vi "Database_FGV.vi"(8 "error in (no error)":errorcluster, 10 "Write DB Data":T1, 11 "DB Control":T3=enum."Open") -> (0 "error out":errorcluster, 3 "DB Data Out":T1)   [LabVIEW 2013]
doc: "The Database FGV provides access to the file/DB components, manages reads and writes, and provides default data when the file/DB is not available."
uses:
  DB_Data.ctl
  Error Handler/Error_Control.ctl
  Controller/Hardware_Enum.ctl
  DB_control.ctl
panel:
  # "[Covers: CD1A]"
  # "[Covers: CD1B]"
  # "[Covers: CD1C]"
  # "[Covers: CD1D]"
  # "Used for Hardware change over"
  # "[Covers: CD1A]"
  # "[Covers: CD1B]"
  # "[Covers: CD1C]"
  # "[Covers: CD1D]"
  # "Used for Hardware change over"
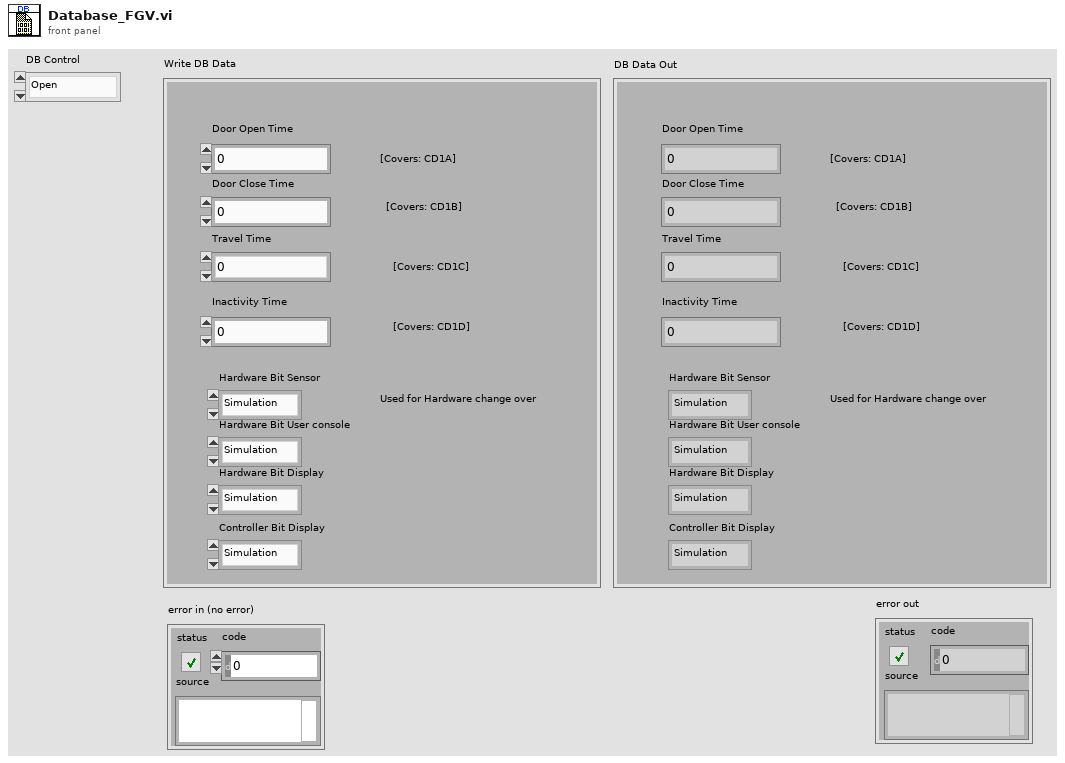
[diagram p1: front panel]
types:
  T1 = typedef "DB_Data.ctl" = cluster{"Door Open Time":dbl, "Travel Time":dbl, "Inactivity Time":dbl, "Door Close Time ":dbl, "Hardware Bit Sensor":T2, "Hardware Bit User console":T2, "Hardware Bit Display":T2, "Controller Bit Display":T2}
  T2 = typedef "Hardware_Enum.ctl" = enum16{"Simulation", "Hardware"}
  T3 = typedef "DB_control.ctl" = enum16{"Initi_FGV", "Open", "Get_Data", "Write_Data", "Write_File", "Close_File"}
  T4 = typedef "Error_Control.ctl" = enum16{"Init", "Console_err", "Process_err", "Sensor_err"}
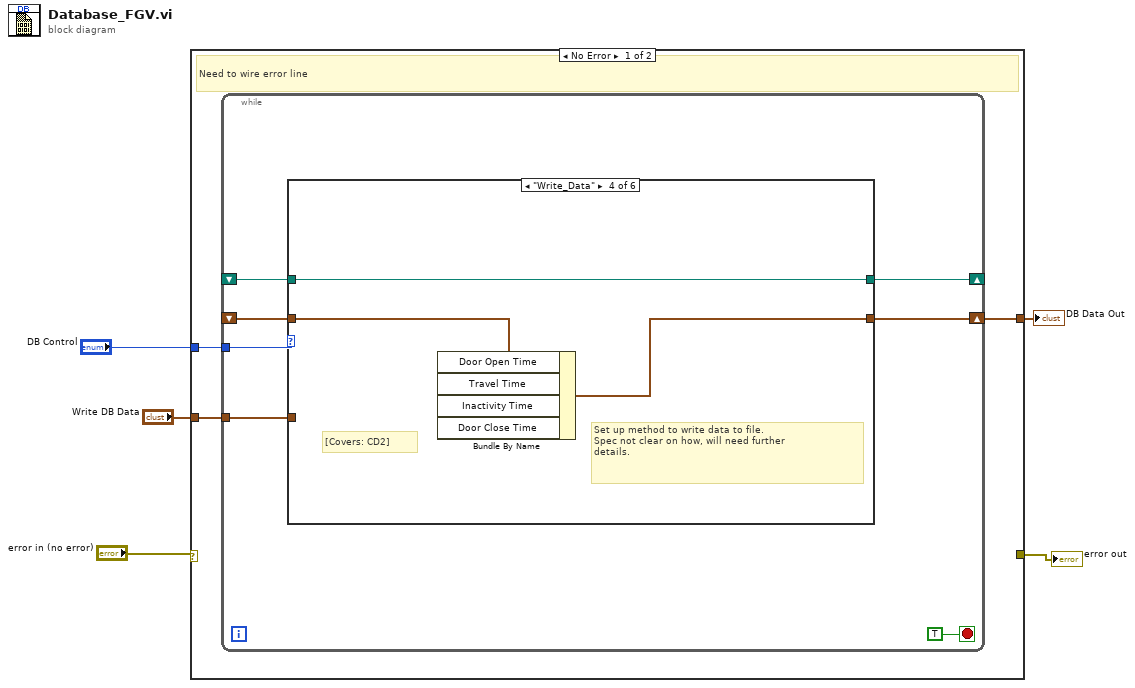
[diagram p0: block diagram]
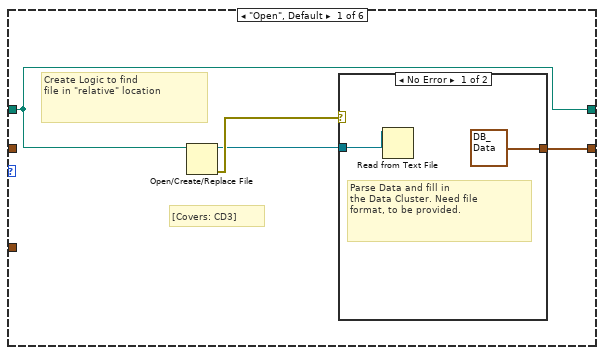
[diagram p2: hidden frame]
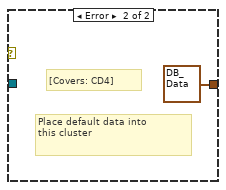
[diagram p3: hidden frame]
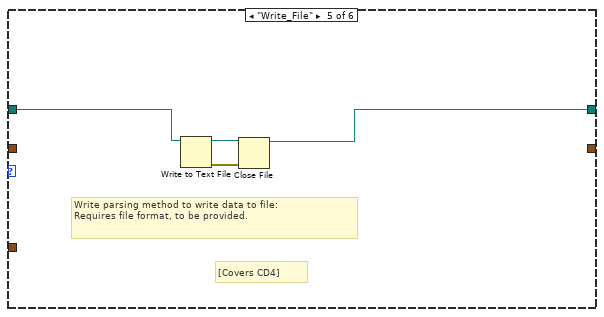
[diagram p6: hidden frame]
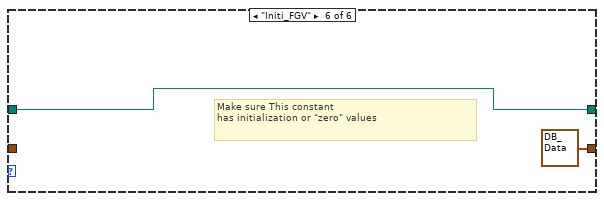
[diagram p7: hidden frame]
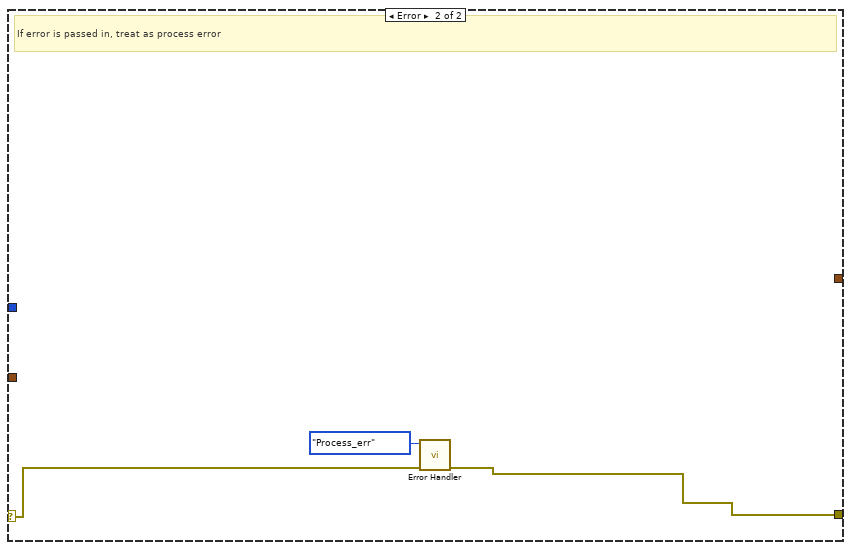
[diagram p8: hidden frame]
diagram:
  n1 = case shown="No Error" "error in (no error)" {
    selector: "error in (no error)" -> [_ w37]
    tunnel: "DB Control" -> [w8 _]
    tunnel: "Write DB Data" -> [w7 _]
    tunnel: [_ w36] -> w2
    tunnel: [w6 _] -> w1
    frame No Error {
      # "Need to wire error line"
      n2 = while {
        tunnel: w8 -> [w14]
        shift-right: [w12] -> w6
        shift-left: _ -> [w11]
        tunnel: w7 -> [w10]
        shift-right: [w9] -> _
        shift-left: _ -> [w13]
        stop <- TRUE stop-if-true
        n3 = case shown="\"Write_Data\"" w14 {
          tunnel: w13 -> [w19 w23 w24 w26 w30 w33]
          tunnel: [w16 _ w25 w27 _ T1 {"Door Open Time"=0.0, "Travel Time"=0.0, "Inactivity Time"=0.0, "Door Close Time "=0.0, "Hardware Bit Sensor"=enum."Simulation", "Hardware Bit User console"=enum."Simulation", "Hardware Bit Display"=enum."Simulation", "Controller Bit Display"=enum."Simulation"} ("DB Data")] -> w12
          tunnel: w11 -> [_ _ w25 w28 _ _]
          tunnel: w10 -> [_ _ _ _ _ _]
          tunnel: [w19 w23 w24 w26 w29 w33] -> w9
          frame "Open", Default {
            # "Create Logic to find\nfile in \"relative\" location"
            # "[Covers: CD3]"
            n4 = Open/Create/Replace File(file path (use dialog)=w19) -> (refnum out=w17:refnum<file>, error out=w18:errorcluster)  [unwired: 5 in, 1 out]
            n5 = case shown="No Error" w18 {
              tunnel: w17 -> [w21 _]
              tunnel: [T1 {"Door Open Time"=0.0, "Travel Time"=0.0, "Inactivity Time"=0.0, "Door Close Time "=0.0, "Hardware Bit Sensor"=enum."Simulation", "Hardware Bit User console"=enum."Simulation", "Hardware Bit Display"=enum."Simulation", "Controller Bit Display"=enum."Simulation"} ("DB Data") T1 {"Door Open Time"=0.0, "Travel Time"=0.0, "Inactivity Time"=0.0, "Door Close Time "=0.0, "Hardware Bit Sensor"=enum."Simulation", "Hardware Bit User console"=enum."Simulation", "Hardware Bit Display"=enum."Simulation", "Controller Bit Display"=enum."Simulation"} ("DB Data")] -> w16
              frame No Error {
                # "Parse Data and fill in \nthe Data Cluster. Need file \nformat, to be provided."
                n6 = Read from Text File(file (use dialog)=w21) -> ()  [unwired: 3 in, 4 out]
              }
              frame Error {
                # "[Covers: CD4]"
                # "Place default data into\nthis cluster"
              }
            }
          }
          frame "Close_File" {
            # "Close file here."
          }
          frame "Get_Data" {
            # "Just pass data for read."
            # "[Covers: CD4]"
          }
          frame "Write_Data" {
            # "Set up method to write data to file.  \nSpec not clear on how, will need further \ndetails."
            # "[Covers: CD2]"
            n7 = Bundle By Name(cluster=w28) -> (w27:T1)  [unwired: 4 in]
          }
          frame "Write_File" {
            # "[Covers CD4]"
            # "Write parsing method to write data to file:\nRequires file format, to be provided."
            n8 = Write to Text File(file (use dialog)=w30) -> (refnum out=w31:refnum<file>, error out=w32:errorcluster)  [unwired: 3 in, 1 out]
            n9 = Close File(refnum=w31, error in=w32) -> (path=w29:path)  [unwired: 1 out]
          }
          frame "Initi_FGV" {
            # "Make sure This constant \nhas initialization or \"zero\" values"
          }
        }
      }
    }
    frame Error {
      # "If error is passed in, treat as process error"
      n10 = call "Error Handler.vi"("error in (no error)"=w37, "Error_Control"=Error_Control."Process_err") -> ("error out"=w36:errorcluster)  [unwired: 9 in]
    }
  }
  "error out" <- w2
  "DB Data Out" <- w1
